vi "Substract(CDB[]).vi"(1 "Enable(T)":bool=TRUE, 2 "In":cdb[](array[numeric]), 4 "n":cdb=1.0+0.0i) -> (6 "Out":cdb[](array[numeric]) format="%.2f")   [LabVIEW 2013]
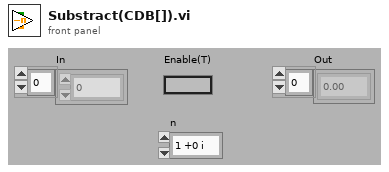
[diagram p1: front panel]
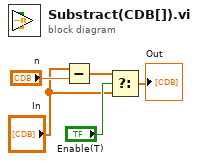
[diagram p0: block diagram]
diagram:
  n1 = Subtract(x="In", y="n") -> (x-y=w1:cdb[])
  n2 = Select(t=w1, s="Enable(T)", f="In") -> (s? t:f=→"Out":cdb[])
